vi "RT Main.vi"() -> ()   [LabVIEW 2024]
uses:
  Shared Modules/CAN Commands Interpreter/CAN Frame Data.ctl
  Shared Modules/CAN Commands Interpreter/XNET Session Settings.ctl
  Type Definitions/ECU States.ctl
  <vilib>/userDefined/High Color/nirio_resource_hc.ctl
  Shared Modules/CAN Commands Interpreter/Command Values.ctl
  Modules/ECU Internal Communications/Notifiers - Create.vi
  Modules/ECU Internal Communications/Queues - Create.vi
  Shared Modules/CAN Commands Interpreter/Target Sessions - Initialize Input Session.vi
  Shared Modules/CAN Commands Interpreter/Target Sessions - Initialize Output Session.vi
  Modules/ECU Internal Communications/Notifiers - Get.vi
  Shared Modules/CAN Commands Interpreter/Target Sessions - Stop Session.vi
  Shared Modules/CAN Commands Interpreter/Target Sessions - Start Session.vi
  Shared Modules/CAN Commands Interpreter/Target Sessions - Clear Session.vi
  Modules/ECU Internal Communications/Queues - Destroy.vi
  Modules/ECU Internal Communications/Notifiers - Destroy.vi
  Modules/FPGA RT Interface/FPGA Reference - Close.vi
  Shared Modules/CAN Commands Interpreter/CAN Commands.lvlib
  Modules/ECU Internal Communications/ECU InterComm.lvlib
  Modules/Real-Time ECU/RT Management.lvlib
  Modules/FPGA RT Interface/FPGA Interface.lvlib
panel:
  in  "Tab Control":enum32{"Monitor", "Session Settings", "Errors"}(tab)
  out "Tester Read Data":T1[](array[typedef])=[{"Command"="Release ECU", "XNET Frame"="Tester_Requests\nCAN Dataframes.CAN_Frames", "Payload"=[255, 255, 0, 0, 0, 0, 0, 0], "ID"=1281, "Time Stamp"=timestamp(3796178359.1687856 s since 1904-01-01)}, {"Command"="IDLE", "XNET Frame"="HeartBit\nCAN Dataframes.CAN_Frames", "Payload"=[0, 255, 0, 0, 0, 0, 0, 0], "ID"=1280, "Time Stamp"=timestamp(3796178311.9860034 s since 1904-01-01)}] {"ID" format="%01x"; "Payload" format="%02x"}
  in  "STOP":bool
  out "Current ECU State":T2
  out "Normal Mode Values":fxp<+,18,3>[](array[numeric]) format="%#.3g"
  in  "ECU Sessions":T3[][](array[typedef])=[[{"Interface"="CAN1", "Frame List"=["Tester_Requests\nCAN Dataframes", "HeartBit\nCAN Dataframes"], "Session ID"="", "Session Name"="ECU - Read Tester Requests"}, {"Interface"="CAN1", "Frame List"=["ECU_Responses\nCAN Dataframes"], "Session ID"="", "Session Name"="ECU - Write ECU Responses"}, {"Interface"="CAN1", "Frame List"=["HeartBit\nCAN Dataframes"], "Session ID"="", "Session Name"="ECU - Write Hertbit"}], [{"Interface"="CAN1", "Frame List"=["Crank_Angle\nCAN Dataframes"], "Session ID"="", "Session Name"="ECU - Write Crank Angle"}, {"Interface"="CAN1", "Frame List"=["Throttle\nCAN Dataframes"], "Session ID"="", "Session Name"="ECU - Write Throttle"}, {"Interface"="", "Frame List"=[], "Session ID"="", "Session Name"=""}]]
  out "XNET Read Errors":errorcluster
  out "Main Error":errorcluster
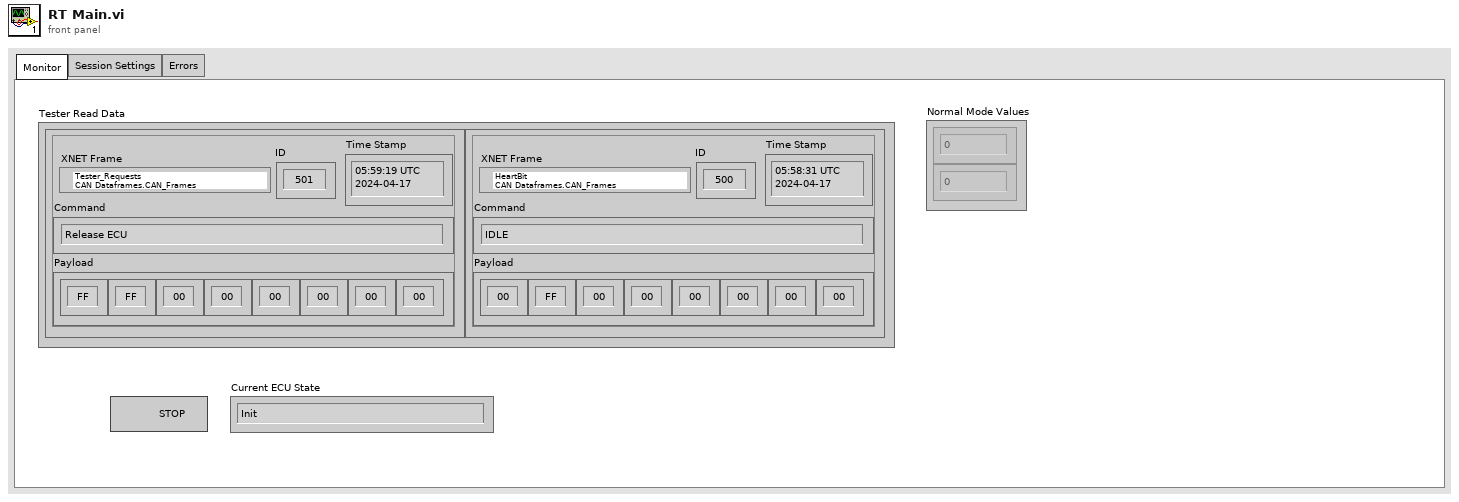
[diagram p1: front panel]
types:
  T1 = typedef "CAN Commands.lvlib/CAN Frame Data.ctl" = cluster{"Command":string, "XNET Frame":refnum<k21>, "Payload":u8[], "ID":u32, "Time Stamp":timestamp}
  T2 = typedef "ECU States.ctl" = enum16{"Init", "Waiting for Tester", "Set Normal Mode", "Run Normal Mode", "Set Manufacturing Mode", "Run Manufacturing Mode", "Restart", "End"}
  T3 = typedef "CAN Commands.lvlib/XNET Session Settings.ctl" = cluster{"Interface":refnum<k21>, "Frame List":refnum<k21>[], "Session ID":refnum<k21>, "Session Name":string}
  T4 = typedef "nirio_resource_hc.ctl" = tag
  T5 = typedef "CAN Commands.lvlib/Command Values.ctl" = cluster{"Command":string, "Value":dbl}
  T6 = typedef "ECU InterComm.lvlib/ECU Notifiers.ctl" = cluster{"Tester Detected":refnum<notifier>, "STOP Reading":refnum<notifier>}
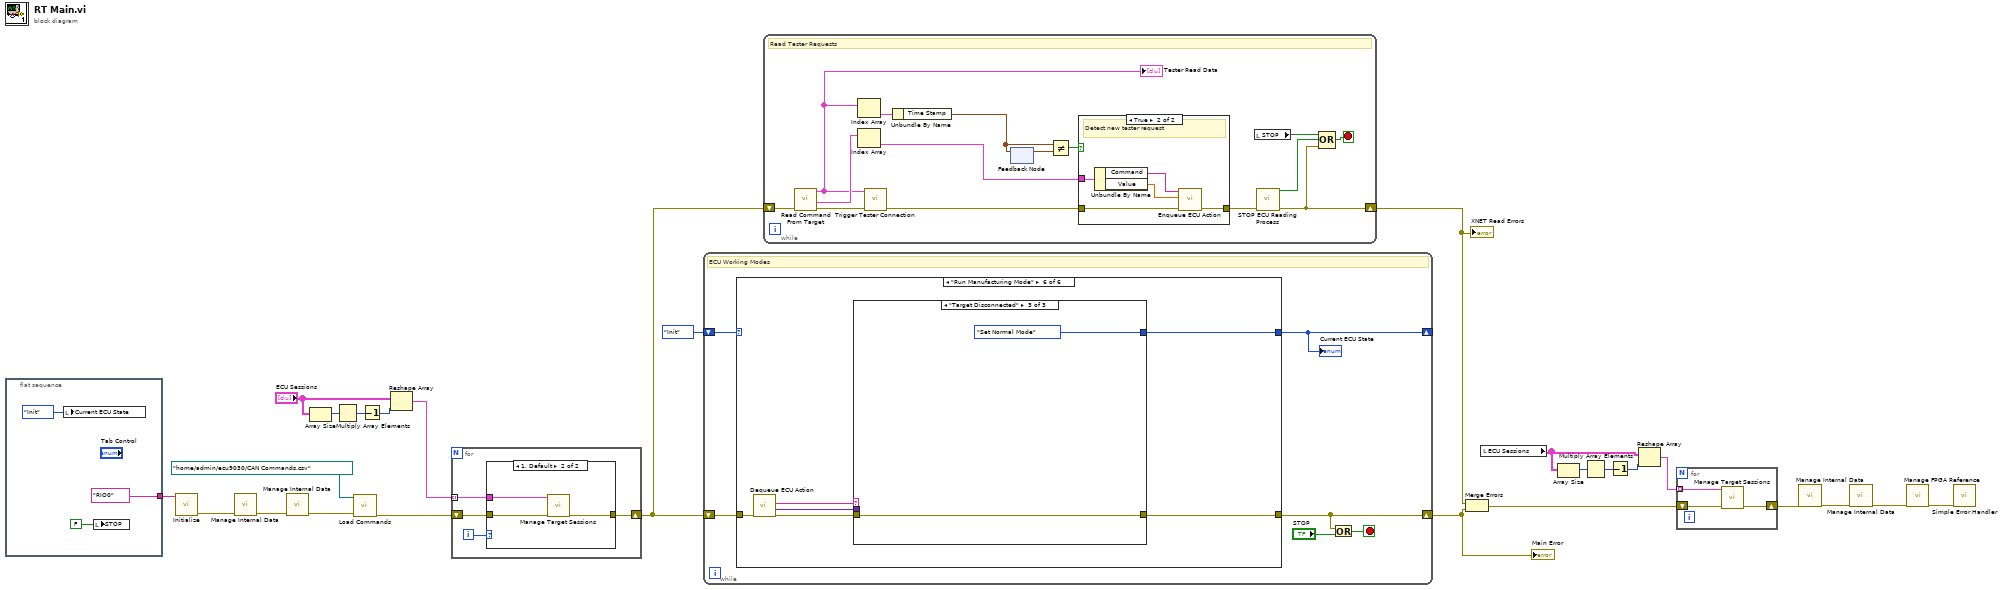
[diagram p0: block diagram]
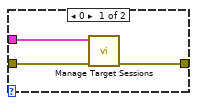
[diagram p2: hidden frame]
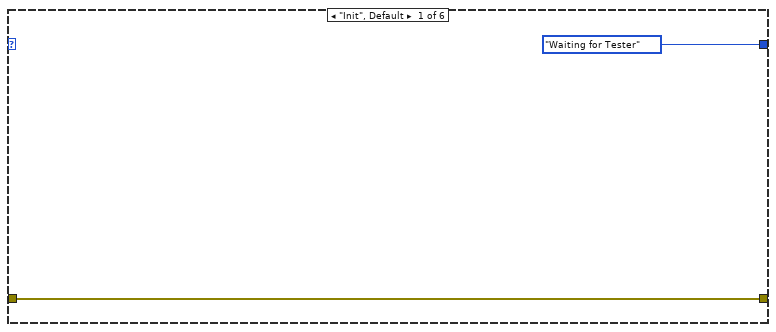
[diagram p3: hidden frame]
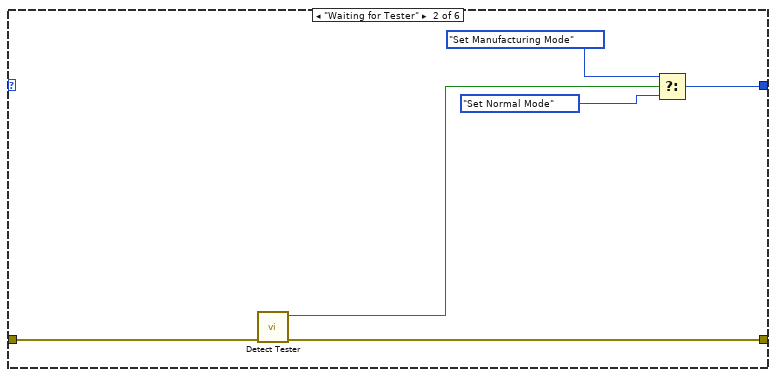
[diagram p4: hidden frame]
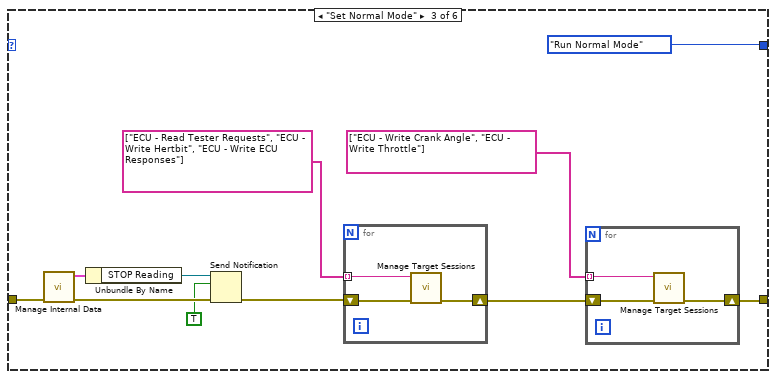
[diagram p5: hidden frame]
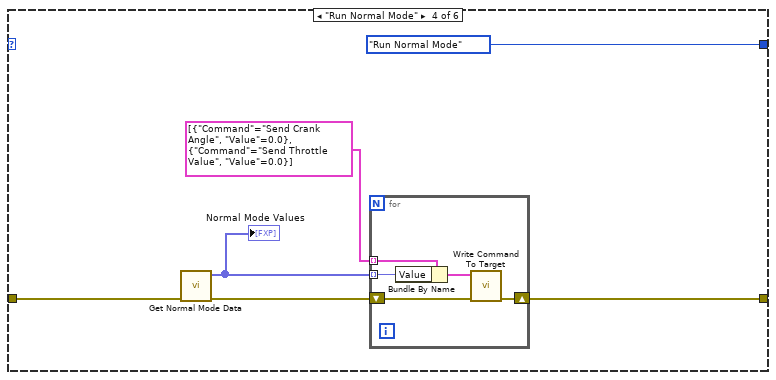
[diagram p6: hidden frame]
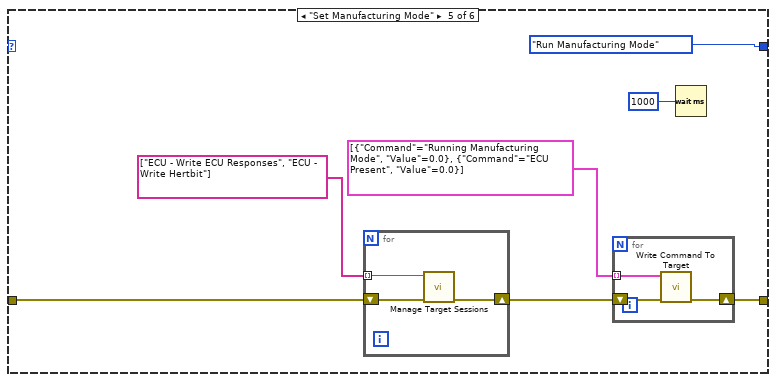
[diagram p7: hidden frame]
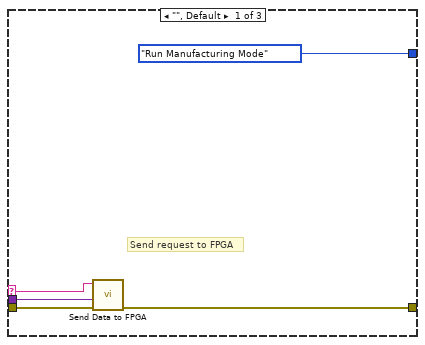
[diagram p8: hidden frame]
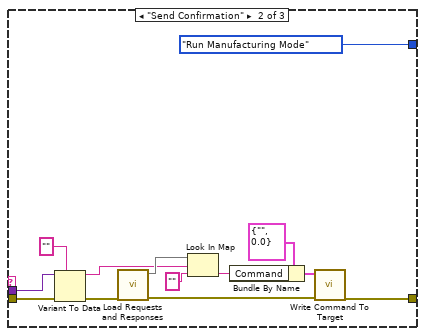
[diagram p9: hidden frame]
diagram:
  n1 = flat-sequence {
    tunnel: [T4 "RIO0" ("FPGA resource name")] -> w16
    frame #0 {
      n2 = local write "Current ECU State"(ECU_States."Init" ("Enum")) -> ()
      n3 = local write "STOP"(FALSE ("STOP")) -> ()
    }
  }
  n4 = call "Initialize.vi"("FPGA resource name"=w16) -> ("error out"=w17:errorcluster)  [unwired: 9 in, 1 out]
  n5 = call-poly "Manage Internal Data.vi"("error in"=w17) -> ("error out"=w21:errorcluster)  [unwired: 10 in]
  n6 = call-poly "Manage Internal Data.vi"("error in"=w21) -> ("error out"=w22:errorcluster)  [unwired: 10 in]
  n7 = Array Size(array="ECU Sessions") -> (size(s)=w11:i32[])
  n8 = Multiply Array Elements(1:w11) -> (0:w10:i32)
  n9 = call "Load Commands.vi"("error in"=w22, "Commands File (CSV)"=path "/home/admin/ecu9030/CAN Commands.csv") -> ("error out"=w18:errorcluster)  [unwired: 9 in]
  n10 = Decrement(x=w10) -> (x-1=w8:i32)
  n11 = Reshape Array("ECU Sessions", w8) -> (w7:T3[])
  n12 = for {
    shift-right: [w31] -> w12
    shift-left: w18 -> [w32]
    tunnel: w7 -> [w29] mode=indexing
    i -> [w30]
    n13 = case shown="1, Default" w30 {
      tunnel: w32 -> [w34 w38]
      tunnel: [w35 w37] -> w31
      tunnel: w29 -> [w33 w36]
      frame 0 {
        n14 = call-poly "Manage Target Sessions.vi"("error in"=w34, "XNET Session Resouces"=w33) -> ("error out"=w35:errorcluster)  [unwired: 9 in]
      }
      frame 1, Default {
        n15 = call-poly "Manage Target Sessions.vi"("error in"=w38, "XNET Session Resouces"=w36) -> ("error out"=w37:errorcluster)  [unwired: 9 in]
      }
    }
  }
  n16 = while {
    shift-right: [w41] -> w15
    shift-left: w12 -> [w43]
    shift-right: [w40] -> _
    shift-left: ECU_States."Init" ("Enum") -> [w42]
    stop <- w44 stop-if-true
    # "ECU Working Modes"
    n17 = case shown="\"Run Manufacturing Mode\"" w42 {
      tunnel: w43 -> [w46 w49 w58 w71 w83 w96]
      tunnel: [w46 w48 w59 w70 w82 w95] -> w41
      tunnel: [ECU_States."Waiting for Tester" ("Enum") w52 ECU_States."Run Normal Mode" ("Enum") ECU_States."Run Normal Mode" ("Enum") ECU_States."Run Manufacturing Mode" ("Enum") w94] -> w40
      frame "Init", Default {
      }
      frame "Waiting for Tester" {
        n18 = call "Detect Tester.vi"("error in"=w49) -> ("error out"=w48:errorcluster, "Tester Detected"=w47:bool)  [unwired: 9 in]
        n19 = Select(t=ECU_States."Set Manufacturing Mode" ("Enum"), s=w47, f=ECU_States."Set Normal Mode" ("Enum")) -> (s? t:f=w52:T2)
      }
      frame "Set Normal Mode" {
        n20 = call-poly "Manage Internal Data.vi"("error in"=w58) -> ("error out"=w57:errorcluster, "ECU Notifiers"=w56:T6)  [unwired: 9 in]
        n21 = Unbundle By Name(w56) -> ("STOP Reading"=w55:refnum<notifier>)
        n22 = Send Notification(notification=TRUE, notifier=w55, error in (no error)=w57) -> (error out=w53:errorcluster)  [unwired: 1 out]
        n23 = for {
          shift-right: [w66] -> w62
          shift-left: w53 -> [w65]
          tunnel: string[] ["ECU - Read Tester Requests", "ECU - Write Hertbit", "ECU - Write ECU Responses"] -> [w64] mode=indexing
          n24 = call-poly "Manage Target Sessions.vi"("error in"=w65, "Session Name"=w64) -> ("error out"=w66:errorcluster)  [unwired: 9 in]
        }
        n25 = for {
          tunnel: string[] ["ECU - Write Crank Angle", "ECU - Write Throttle"] -> [w69] mode=indexing
          shift-right: [w68] -> w59
          shift-left: w62 -> [w67]
          n26 = call-poly "Manage Target Sessions.vi"("error in"=w67, "Session Name"=w69) -> ("error out"=w68:errorcluster)  [unwired: 9 in]
        }
      }
      frame "Run Normal Mode" {
        n27 = call "Get Normal Mode Data.vi"("error in"=w71) -> ("error out"=w74:errorcluster, "Normal Mode Values"=w73:fxp<+,18,3>[])  [unwired: 9 in]
        "Normal Mode Values" <- w73
        n28 = for {
          shift-right: [w79] -> w70
          shift-left: w74 -> [w80]
          tunnel: T5[] [{"Command"="Send Crank Angle", "Value"=0.0}, {"Command"="Send Throttle Value", "Value"=0.0}] -> [w78] mode=indexing
          tunnel: w73 -> [w76] mode=indexing
          n29 = Bundle By Name(cluster=w78, "Value"=w76) -> (w77:T5)
          n30 = call "Write Command To Target.vi"("error out"=w80, "Command"=w77) -> ("error out"=w79:errorcluster)  [unwired: 9 in]
        }
      }
      frame "Set Manufacturing Mode" {
        n31 = for {
          tunnel: string[] ["ECU - Write ECU Responses", "ECU - Write Hertbit"] -> [w93] mode=indexing
          shift-right: [w92] -> w84
          shift-left: w83 -> [w91]
          n32 = call-poly "Manage Target Sessions.vi"("error in"=w91, "Session Name"=w93) -> ("error out"=w92:errorcluster)  [unwired: 9 in]
        }
        n33 = for {
          shift-right: [w89] -> w82
          shift-left: w84 -> [w90]
          tunnel: T5[] [{"Command"="Running Manufacturing Mode", "Value"=0.0}, {"Command"="ECU Present", "Value"=0.0}] -> [w88] mode=indexing
          n34 = call "Write Command To Target.vi"("error out"=w90, "Command"=w88) -> ("error out"=w89:errorcluster)  [unwired: 9 in]
        }
        n35 = Wait (ms)(milliseconds to wait=u32 1000) -> ()  [unwired: 1 out]
      }
      frame "Run Manufacturing Mode" {
        n36 = call "Dequeue ECU Action.vi"("error in"=w96) -> ("error out"=w97:errorcluster, "Data"=w98:variant, "Message"=w99:string)  [unwired: 8 in]
        n37 = case shown="\"Target Disconnected\"" w99 {
          selector: w99 -> [w102 _ _]
          tunnel: [w103 w113 w118] -> w95
          tunnel: w97 -> [w104 w112 w118]
          tunnel: w98 -> [w101 w106 _]
          tunnel: [ECU_States."Run Manufacturing Mode" ("Enum") ECU_States."Run Manufacturing Mode" ("Enum") ECU_States."Set Normal Mode" ("Enum")] -> w94
          frame "", Default {
            # "Send request to FPGA"
            n38 = call "Send Data to FPGA.vi"("error in (no error)"=w104, "Data"=w101, "Command"=w102) -> ("error out"=w103:errorcluster)  [unwired: 8 in]
          }
          frame "Send Confirmation" {
            n39 = Variant To Data(error in=w112, type="" ("default value"), Variant=w106) -> (data=w107:string, error out=w116:errorcluster)
            n40 = call "Load Requests and Responses.vi"("error in (no error)"=w116) -> ("error out"=w114:errorcluster, "Request and Responses In out"=w111:map{string, string})  [unwired: 9 in]
            n41 = Look In Map(map=w111, key=w107, default value="") -> (value=w108:string)  [unwired: 1 out]
            n42 = Bundle By Name(cluster=T5 {"Command"="", "Value"=0.0} ("Command"), "Command"=w108) -> (w109:T5)
            n43 = call "Write Command To Target.vi"("error out"=w114, "Command"=w109) -> ("error out"=w113:errorcluster)  [unwired: 9 in]
          }
          frame "Target Disconnected" {
          }
        }
      }
    }
    "Current ECU State" <- w40
    n44 = Or(x=w41, y="STOP") -> (x .or. y?=w44:bool)
  }
  "Main Error" <- w15
  n45 = while {
    shift-right: [w121] -> w24
    shift-left: w12 -> [w133]
    stop <- w134 stop-if-true
    # "Read Tester Requests"
    n46 = call "Read Command From Target.vi"("error in"=w133) -> ("error out"=w132:errorcluster, "Commands"=w128:T5[], "XNET Data"=w127:T1[])  [unwired: 7 in, 1 out]
    "Tester Read Data" <- w127
    n47 = Index Array(array=w127) -> (element=w126:T1)  [unwired: 1 in]
    n48 = Index Array(array=w128) -> (element=w129:T5)  [unwired: 1 in]
    n49 = call "Trigger Tester Connection.vi"("error in"=w132, "ECU Read Data"=w127) -> ("error out"=w131:errorcluster)  [unwired: 9 in]
    n50 = Unbundle By Name(w126) -> ("Time Stamp"=w125:timestamp)
    n51 = feedback-in #1(w125) -> ()
    n52 = feedback #1() -> (w130:timestamp)  [unwired: 1 in]
    n53 = Not Equal?(x=w125, y=w130) -> (x != y?=w124:bool)
    n54 = case shown="True" w124 {
      tunnel: w131 -> [w135 w140]
      tunnel: [w135 w139] -> w123
      tunnel: w129 -> [_ w138]
      frame False {
      }
      frame True {
        # "Detect new tester request"
        n55 = Unbundle By Name(w138) -> ("Command"=w137:string, "Value"=w136:dbl)
        n56 = call "Enqueue ECU Action.vi"("error in"=w140, "Command"=w136, "Message"=w137) -> ("error out"=w139:errorcluster)  [unwired: 8 in]
      }
    }
    n57 = local read "STOP"() -> (w120:bool)
    n58 = call "STOP ECU Reading Process.vi"("error in"=w123) -> ("error out"=w121:errorcluster, "End of Communication"=w122:bool)  [unwired: 9 in]
    n59 = Compound Arithmetic op=OR(w120, w122, w121) -> (w134:bool)
  }
  "XNET Read Errors" <- w24
  n60 = Merge Errors(w24, w15) -> (w25:errorcluster)
  n61 = local read "ECU Sessions"() -> (w3:T3[][])
  n62 = Array Size(array=w3) -> (size(s)=w4:i32[])
  n63 = Multiply Array Elements(1:w4) -> (0:w5:i32)
  n64 = Decrement(x=w5) -> (x-1=w6:i32)
  n65 = Reshape Array(w3, w6) -> (w1:T3[])
  n66 = for {
    shift-right: [w142] -> w20
    shift-left: w25 -> [w143]
    tunnel: w1 -> [w141] mode=indexing
    n67 = call-poly "Manage Target Sessions.vi"("error in"=w143, "XNET Session"=w141) -> ("error out"=w142:errorcluster)  [unwired: 9 in]
  }
  n68 = call-poly "Manage Internal Data.vi"("error in"=w20) -> ("error out"=w19:errorcluster)  [unwired: 10 in]
  n69 = call-poly "Manage Internal Data.vi"("error in"=w19) -> ("error out"=w14:errorcluster)  [unwired: 10 in]
  n70 = call-poly "Manage FPGA Reference.vi"("error in"=w14) -> ("error out"=w13:errorcluster)  [unwired: 10 in]
  n71 = call <vilib>:"Simple Error Handler.vi"("error in (no error)"=w13) -> ()  [unwired: 4 in, 5 out]
